vi "Digital Read N Chans.vi"(8 "Error In":errorcluster, 10 "DI Channels":u8[](array[numeric]), 11 "LINX Resource":T1) -> (0 "Error Out":errorcluster, 2 "Values":bool[](array[boolean]), 3 "LINX Resource":T1)   [LabVIEW 2011, in "LMH-LINX.lvlib"]
doc: "Read the values of the specified digital input channels."
uses:
  LMH-LINX.lvlib
  Private/Type Defs/LINX Ref.ctl
  Private/Type Defs/Platform.ctl
  Private/Type Defs/Interface.ctl
  Private/Device/Type Defs/LINX Device Config.ctl
  Private/Device/Type Defs/TCP Config.ctl
  Private/Device/Type Defs/Channels.ctl
  Private/Type Defs/Peripheral.ctl
  Private/myRIO/myRIO.lvlib
  Private/Device/Device.lvlib
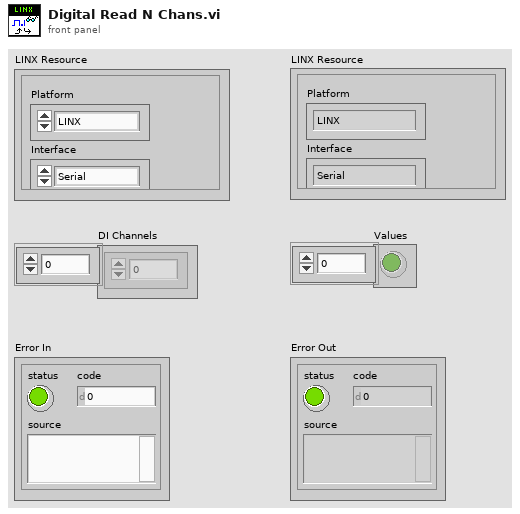
[diagram p1: front panel]
types:
  T1 = typedef "LMH-LINX.lvlib/LINX Ref.ctl" = cluster{"Platform":T2, "Interface":T3, "LINX Device Config":T4}
  T2 = typedef "LMH-LINX.lvlib/Platform.ctl" = enum16{"LINX", "myRIO"}
  T3 = typedef "LMH-LINX.lvlib/Interface.ctl" = enum16{"Serial", "TCP"}
  T4 = typedef "LMH-LINX.lvlib/Device.lvlib/LINX Device Config.ctl" = cluster{"Interface":T3, "COM Port":refnum<visa-resource-name>, "TCP Configuration":T5, "Device Family":u8, "Device ID":u8, "Device Name":string, "TCP Ref":refnum<k5>, "Channels":T6}
  T5 = typedef "LMH-LINX.lvlib/Device.lvlib/TCP Config.ctl" = cluster{"IP Address":string, "Port":u16}
  T6 = typedef "LMH-LINX.lvlib/Channels.ctl" = cluster{"DI":u8[], "DO":u8[], "AI":u8[], "AO":u8[], "PWM":u8[], "QE":u8[], "UART":u8[], "I2C 2":u8[], "SPI":u8[], "CAN":u8[], "Servo":u8[], "AI Ref (V)":dbl, "AO Ref (V)":dbl, "AO Resolution (Bits)":u8}
  T7 = typedef "LMH-LINX.lvlib/Peripheral.ctl" = enum8{"DI", "DO", "AI", "AO", "PWM", "QE", "UART", "I2C", "SPI", "CAN", "Servo"}
  T8 = typedef "DIO.lvlib/DIO Reference.ctl" = cluster{"myRIO Reference":T9, "DIO Channels List":T13}
  T9 = typedef "myRIO Generic Hardware Reference.ctl" = cluster{"myRIO Model":T10, "myRIO Hardware Reference":T11}
  T10 = typedef "Hardware Version Enum.ctl" = enum16{"Unknown", "myRIO-1900", "myRIO-1950"}
  T11 = typedef "myRIO v1.0 Reference.ctl" = cluster{"Generic FPGA Reference":T12, "Allow multiple opens":bool}
  T12 = typedef "Generic FPGA Reference.ctl" = refnum<k20>
  T13 = typedef "DIO Channels List.ctl" = T14[]
  T14 = typedef "DIO Channels Enum.ctl" = enum16{"Not Connected", "C/DIO0", "C/DIO1", "C/DIO2", "C/DIO3", "C/DIO4", "C/DIO5", "C/DIO6", "C/DIO7", "A/DIO0", "A/DIO1", "A/DIO2", "A/DIO3", "A/DIO4", "A/DIO5", "A/DIO6", "A/DIO7", "A/DIO8", "A/DIO9", "A/DIO10", "A/DIO11", "A/DIO12", "A/DIO13", "A/DIO14", "A/DIO15", "B/DIO0", "B/DIO1", "B/DIO2", "B/DIO3", "B/DIO4", "B/DIO5", "B/DIO6", "B/DIO7", "B/DIO8", "B/DIO9", "B/DIO10", "B/DIO11", "B/DIO12", "B/DIO13", "B/DIO14", "B/DIO15", "LED0", "LED1", "LED2", "LED3", "Button0"}
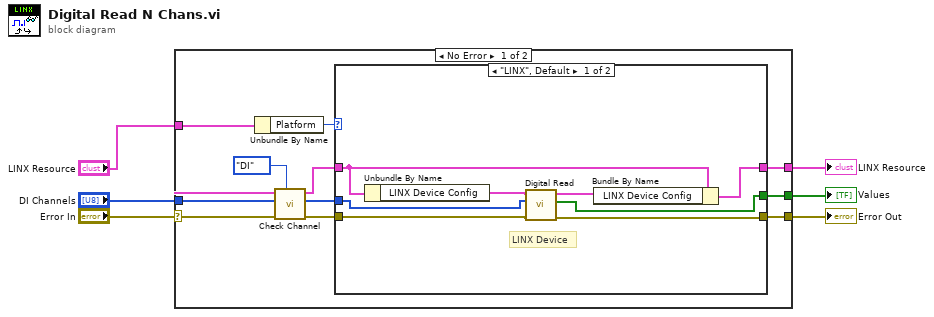
[diagram p0: block diagram]
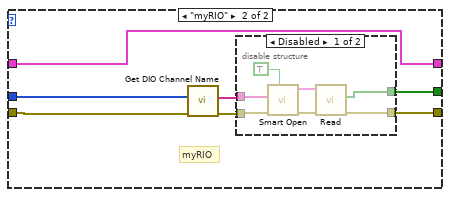
[diagram p2: hidden frame]
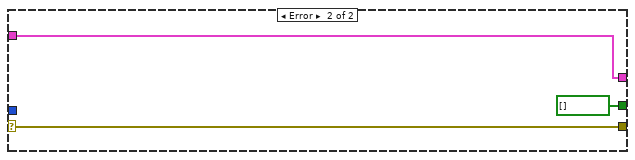
[diagram p4: hidden frame]
diagram:
  n1 = case shown="No Error" "Error In" {
    selector: "Error In" -> [w7 w42]
    tunnel: [w16 w42] -> w6
    tunnel: [w15 w40] -> w5
    tunnel: [w14 bool[] [] ("Values")] -> w4
    tunnel: "LINX Resource" -> [w9 w40]
    tunnel: "DI Channels" -> [w8 _]
    frame No Error {
      n2 = Unbundle By Name(w9) -> ("Platform"=w17:T2)
      n3 = call "Check Channel.vi"("Peripheral"=Peripheral."DI", "Error In"=w7, "Channels"=w8, "LINX Resource"=w9) -> ("Error Out"=w13:errorcluster, "Channels"=w12:u8[], "LINX Resource"=w10:T1)  [unwired: 5 in]
      n4 = case shown="\"LINX\", Default" w17 {
        tunnel: w13 -> [w23 w29]
        tunnel: w10 -> [w25 w32]
        tunnel: [w22 w31] -> w16
        tunnel: [w24 w32] -> w15
        tunnel: w12 -> [w19 w26]
        tunnel: [w18 w30] -> w14
        frame "LINX", Default {
          # "LINX Device"
          n5 = Unbundle By Name(w25) -> ("LINX Device Config"=w20:T4)
          n6 = call "Digital Read.vi"("Error In"=w23, "DIO Channels"=w19, "LINX Device Config"=w20) -> ("Error Out"=w22:errorcluster, "Values"=w18:bool[], "LINX Device Config"=w21:T4)  [unwired: 6 in]
          n7 = Bundle By Name(cluster=w25, "LINX Device Config"=w21) -> (w24:T1)
        }
        frame "myRIO" {
          # "myRIO"
          n8 = call "Get DIO Channel Name.vi"("Error In"=w29, "DIO Channel Nums"=w26) -> ("Error Out"=w28:errorcluster, "DIO Channels"=w27:string[])  [unwired: 8 in]
          n9 = disable-structure shown="Disabled" {
            disable-tunnel: [w39 _] -> w31
            disable-tunnel: w28 -> [w36 _]
            disable-tunnel: w27 -> [w37 _]
            disable-tunnel: [w38 _] -> w30
            frame Disabled {
              n10 = call <vilib>:"Smart Open.vi"("Allow multiple opens?"=TRUE, "error in (no error)"=w36, "Channel Names"=w37) -> ("error out"=w35:errorcluster, "DIO Ref Out"=w34:T8)  [unwired: 7 in]
              n11 = call <vilib>:"Read.vi"("error in (no error)"=w35, "DIO Ref In"=w34) -> ("error out"=w39:errorcluster, "Values"=w38:bool[])  [unwired: 7 in, 1 out]
            }
            frame Enabled {
            }
          }
        }
      }
    }
    frame Error {
    }
  }
  "Error Out" <- w6
  "LINX Resource" <- w5
  "Values" <- w4
